vi "programacionparalela.vi"() -> ()   [LabVIEW 2020]
panel:
  out "Thermometer 12":u8(slide) scale=0.0..100.0
  out "Thermometer 11":u8(slide) scale=0.0..100.0
  out "Thermometer 10":u8(slide) scale=0.0..100.0
  out "Thermometer 9":u8(slide) scale=0.0..100.0
  out "Thermometer 8":u8(slide) scale=0.0..100.0
  out "Thermometer 7":u8(slide) scale=0.0..100.0
  out "Thermometer 6":u8(slide) scale=0.0..100.0
  out "Thermometer 5":u8(slide) scale=0.0..100.0
  out "Thermometer 4":u8(slide) scale=0.0..100.0
  out "Thermometer 3":u8(slide) scale=0.0..100.0
  out "Thermometer 2":u8(slide) scale=0.0..100.0
  out "Thermometer":u8(slide) scale=0.0..100.0
  # "Programacion paralela en labview"
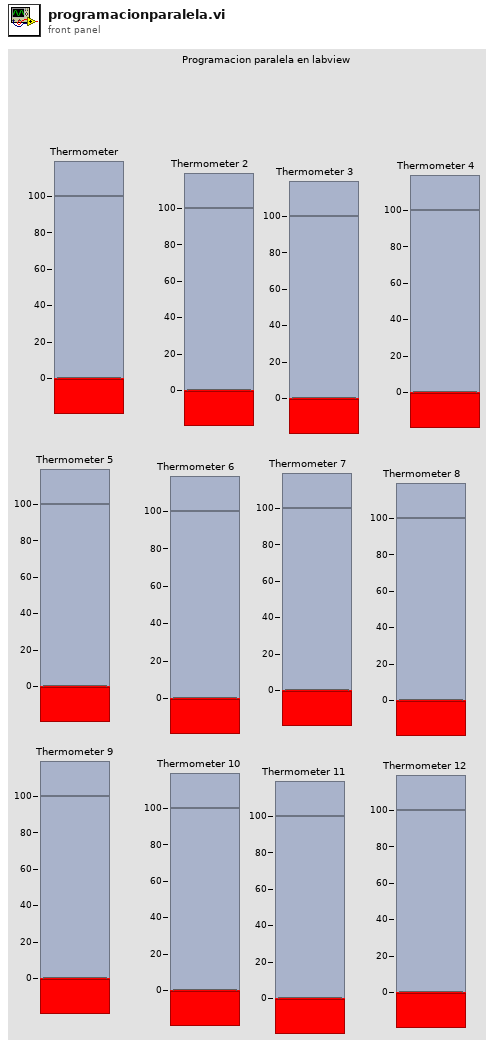
[diagram p1: front panel]
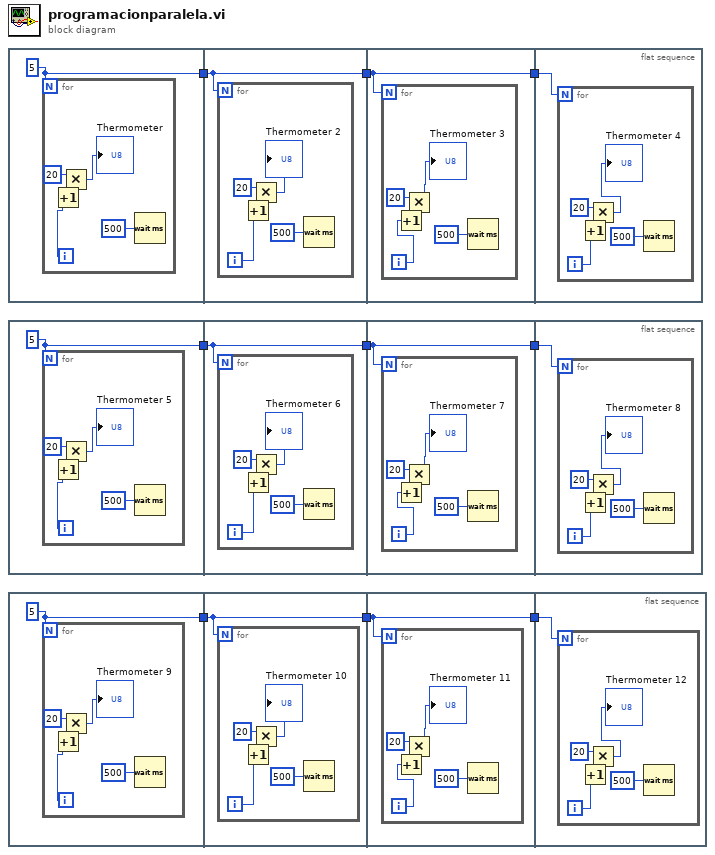
[diagram p0: block diagram]
diagram:
  n1 = flat-sequence {
    tunnel: [w10] -> w9
    tunnel: [w16] -> w8
    tunnel: w9 -> [w16]
    tunnel: [w22] -> w7
    tunnel: w8 -> [w22]
    tunnel: w7 -> [w28]
    frame #0 {
      w10 = 5
      n2 = for {
        N: w10 -> [_]
        i -> [w14]
        n3 = Increment(x=w14) -> (x+1=w12:i32)
        n4 = Multiply(x=20, y=w12) -> (x*y=→"Thermometer":i32)
        n5 = Wait (ms)(milliseconds to wait=u32 500) -> ()  [unwired: 1 out]
      }
    }
    frame #1 {
      n6 = for {
        N: w16 -> [_]
        i -> [w18]
        n7 = Increment(x=w18) -> (x+1=w20:i32)
        n8 = Multiply(x=20, y=w20) -> (x*y=→"Thermometer 2":i32)
        n9 = Wait (ms)(milliseconds to wait=u32 500) -> ()  [unwired: 1 out]
      }
    }
    frame #2 {
      n10 = for {
        N: w22 -> [_]
        i -> [w24]
        n11 = Increment(x=w24) -> (x+1=w26:i32)
        n12 = Multiply(x=20, y=w26) -> (x*y=→"Thermometer 3":i32)
        n13 = Wait (ms)(milliseconds to wait=u32 500) -> ()  [unwired: 1 out]
      }
    }
    frame #3 {
      n14 = for {
        N: w28 -> [_]
        i -> [w30]
        n15 = Increment(x=w30) -> (x+1=w32:i32)
        n16 = Multiply(x=20, y=w32) -> (x*y=→"Thermometer 4":i32)
        n17 = Wait (ms)(milliseconds to wait=u32 500) -> ()  [unwired: 1 out]
      }
    }
  }
  n18 = flat-sequence {
    tunnel: [w34] -> w6
    tunnel: [w40] -> w5
    tunnel: w6 -> [w40]
    tunnel: [w46] -> w4
    tunnel: w5 -> [w46]
    tunnel: w4 -> [w52]
    frame #0 {
      w34 = 5
      n19 = for {
        N: w34 -> [_]
        i -> [w38]
        n20 = Increment(x=w38) -> (x+1=w36:i32)
        n21 = Multiply(x=20, y=w36) -> (x*y=→"Thermometer 5":i32)
        n22 = Wait (ms)(milliseconds to wait=u32 500) -> ()  [unwired: 1 out]
      }
    }
    frame #1 {
      n23 = for {
        N: w40 -> [_]
        i -> [w42]
        n24 = Increment(x=w42) -> (x+1=w44:i32)
        n25 = Multiply(x=20, y=w44) -> (x*y=→"Thermometer 6":i32)
        n26 = Wait (ms)(milliseconds to wait=u32 500) -> ()  [unwired: 1 out]
      }
    }
    frame #2 {
      n27 = for {
        N: w46 -> [_]
        i -> [w48]
        n28 = Increment(x=w48) -> (x+1=w50:i32)
        n29 = Multiply(x=20, y=w50) -> (x*y=→"Thermometer 7":i32)
        n30 = Wait (ms)(milliseconds to wait=u32 500) -> ()  [unwired: 1 out]
      }
    }
    frame #3 {
      n31 = for {
        N: w52 -> [_]
        i -> [w55]
        n32 = Increment(x=w55) -> (x+1=w57:i32)
        n33 = Multiply(x=20, y=w57) -> (x*y=→"Thermometer 8":i32)
        n34 = Wait (ms)(milliseconds to wait=u32 500) -> ()  [unwired: 1 out]
      }
    }
  }
  n35 = flat-sequence {
    tunnel: [w58] -> w3
    tunnel: [w64] -> w2
    tunnel: w3 -> [w64]
    tunnel: [w70] -> w1
    tunnel: w2 -> [w70]
    tunnel: w1 -> [w76]
    frame #0 {
      w58 = 5
      n36 = for {
        N: w58 -> [_]
        i -> [w62]
        n37 = Increment(x=w62) -> (x+1=w60:i32)
        n38 = Multiply(x=20, y=w60) -> (x*y=→"Thermometer 9":i32)
        n39 = Wait (ms)(milliseconds to wait=u32 500) -> ()  [unwired: 1 out]
      }
    }
    frame #1 {
      n40 = for {
        N: w64 -> [_]
        i -> [w66]
        n41 = Increment(x=w66) -> (x+1=w68:i32)
        n42 = Multiply(x=20, y=w68) -> (x*y=→"Thermometer 10":i32)
        n43 = Wait (ms)(milliseconds to wait=u32 500) -> ()  [unwired: 1 out]
      }
    }
    frame #2 {
      n44 = for {
        N: w70 -> [_]
        i -> [w72]
        n45 = Increment(x=w72) -> (x+1=w74:i32)
        n46 = Multiply(x=20, y=w74) -> (x*y=→"Thermometer 11":i32)
        n47 = Wait (ms)(milliseconds to wait=u32 500) -> ()  [unwired: 1 out]
      }
    }
    frame #3 {
      n48 = for {
        N: w76 -> [_]
        i -> [w78]
        n49 = Increment(x=w78) -> (x+1=w80:i32)
        n50 = Multiply(x=20, y=w80) -> (x*y=→"Thermometer 12":i32)
        n51 = Wait (ms)(milliseconds to wait=u32 500) -> ()  [unwired: 1 out]
      }
    }
  }
